vi "RunSubsystem.vi"(8 "error in (no error)":errorcluster, 11 "AutoDrive in":refnum<class "AutoDrive.lvclass">) -> (0 "error out":errorcluster, 3 "AutoDrive out":refnum<class "AutoDrive.lvclass">)   [LabVIEW 2017, in "AutoDrive.lvclass"]
uses:
  AutoDrive.lvclass
  AutoSubroutine.lvclass
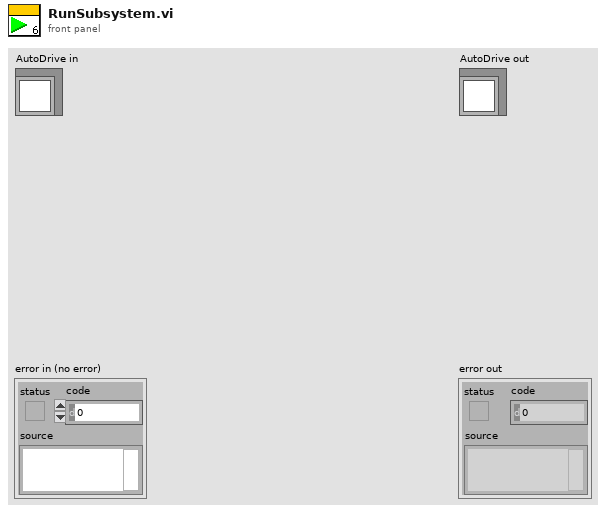
[diagram p1: front panel]
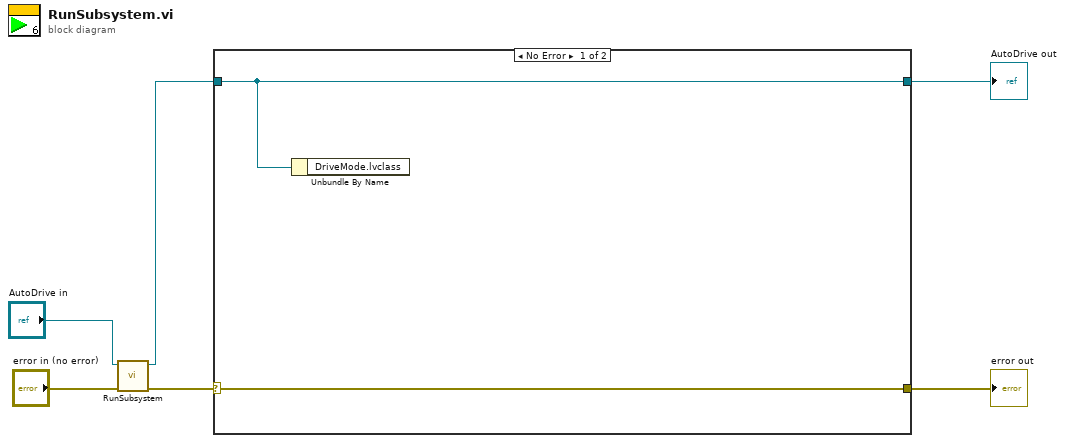
[diagram p0: block diagram]
diagram:
  n1 = call-parent "RunSubsystem.vi"("error in (no error)"="error in (no error)", "AutoSubroutine in"="AutoDrive in") -> ("error out"=w4:errorcluster, "AutoSubroutine out"=w2:refnum<class "AutoDrive.lvclass">)  [unwired: 8 in]
  n2 = case shown="No Error" w4 {
    selector: w4 -> [w8 w9]
    tunnel: [w8 w9] -> w3
    tunnel: w2 -> [w7 w10]
    tunnel: [w7 w10] -> w1
    frame No Error {
      n3 = Unbundle By Name(w7) -> ()  [unwired: 1 out]
    }
    frame Error {
    }
  }
  "error out" <- w3
  "AutoDrive out" <- w1
